vi "Srednia FVG.vi"(6 "Zakres (5)":i32=3, 7 "Akcje (Mean)":T1=enum."Mean", 8 "error in (no error)":errorcluster, 10 "temperatura in":dbl) -> (0 "error out":errorcluster, 2 "temperatura out":dbl, 3 "średnia out":dbl)   [LabVIEW 2013]
doc: "Liczy średnią z pomiarów\nStruktura pliku FVG"
uses:
  inne pliki/Akcje FVG.ctl
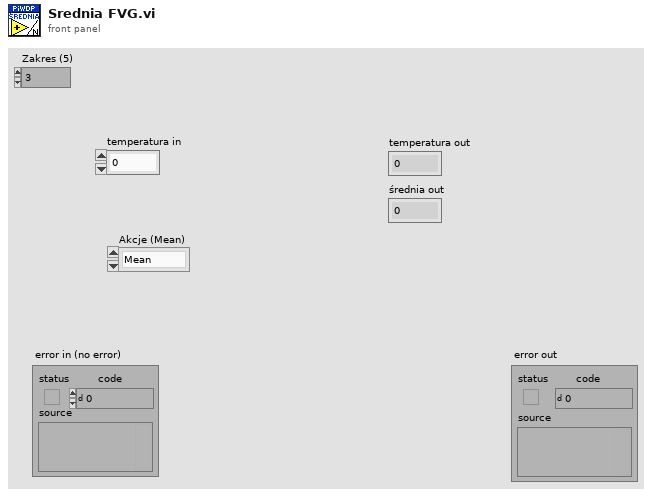
[diagram p1: front panel]
types:
  T1 = typedef "Akcje FVG.ctl" = enum16{"Config", "Mean"}
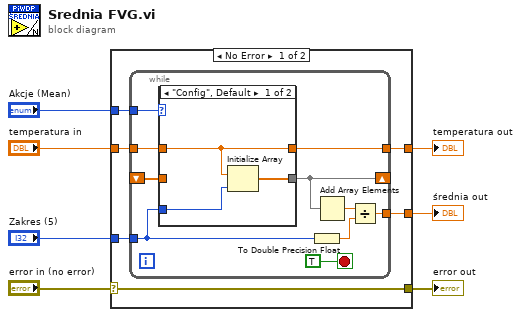
[diagram p0: block diagram]
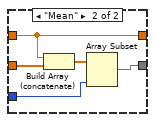
[diagram p2: hidden frame]
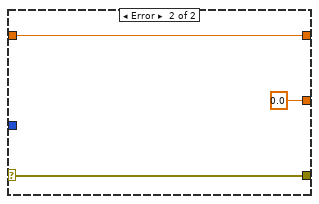
[diagram p3: hidden frame]
diagram:
  n1 = case shown="No Error" "error in (no error)" {
    selector: "error in (no error)" -> [w13 w34]
    tunnel: [w13 w34] -> w6
    tunnel: "temperatura in" -> [w12 w33]
    tunnel: "Zakres (5)" -> [w11 _]
    tunnel: [w10 w33] -> w3
    tunnel: [w8 0.0] -> w2
    tunnel: "Akcje (Mean)" -> [w9 _]
    frame No Error {
      n2 = while {
        tunnel: w12 -> [w21]
        tunnel: w11 -> [w14]
        shift-right: [w15] -> _
        shift-left: _ -> [w22]
        tunnel: [w19] -> w10
        tunnel: w9 -> [w20]
        tunnel: [w16] -> w8
        stop <- TRUE stop-if-true
        n3 = case shown="\"Config\", Default" w20 {
          tunnel: w22 -> [_ w30]
          tunnel: w21 -> [w25 w27]
          tunnel: [w24 w29] -> w15
          tunnel: w14 -> [w26 w28]
          tunnel: [w25 w27] -> w19
          frame "Config", Default {
            n4 = Initialize Array(w25, w26) -> (w24:dbl[])
          }
          frame "Mean" {
            n5 = Build Array (concatenate)(w27, w30) -> (w31:dbl[])
            n6 = Array Subset(array=w31, length=w28) -> (w29:dbl[])  [unwired: 1 in]
          }
        }
        n7 = To Double Precision Float(number=w14) -> (double precision float=w17:dbl)
        n8 = Add Array Elements(numeric array=w15) -> (sum=w18:dbl)
        n9 = Divide(x=w18, y=w17) -> (x/y=w16:dbl)
      }
    }
    frame Error {
    }
  }
  "error out" <- w6
  "temperatura out" <- w3
  "średnia out" <- w2
